vi "TransferFile.vi"(1 "Choose the Destination File Folder (Absolute Path) for AWG's files system":path, 2 "Choose the Source File (Absolute Path)":path, 4 "error in (no error)":errorcluster, 5 "ChunkSize":u32=10000000, 6 "Set File Name (with Extension)":string, 7 "VISA resource name":refnum<visa-resource-name>) -> (0 "error out":errorcluster, 3 "VISA resource name out":refnum<visa-resource-name>)   [LabVIEW 2020, in "Active Technologies AWG3000.lvlib"]
uses:
  Active Technologies AWG3000.lvlib
panel:
  # "Note: for the drive C is allowed transfer a file only to the default folder or to its subdirectories. \nNo limitation for the other drives.\nTo know the default folder, run GetDefaultDriveCFolder.vi."
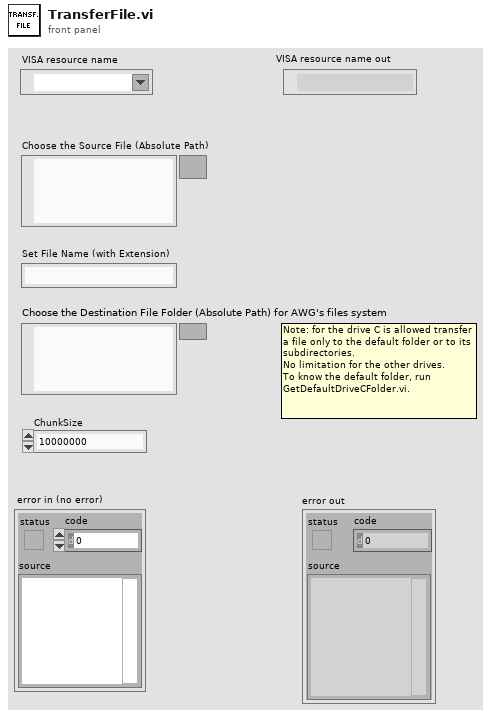
[diagram p1: front panel]
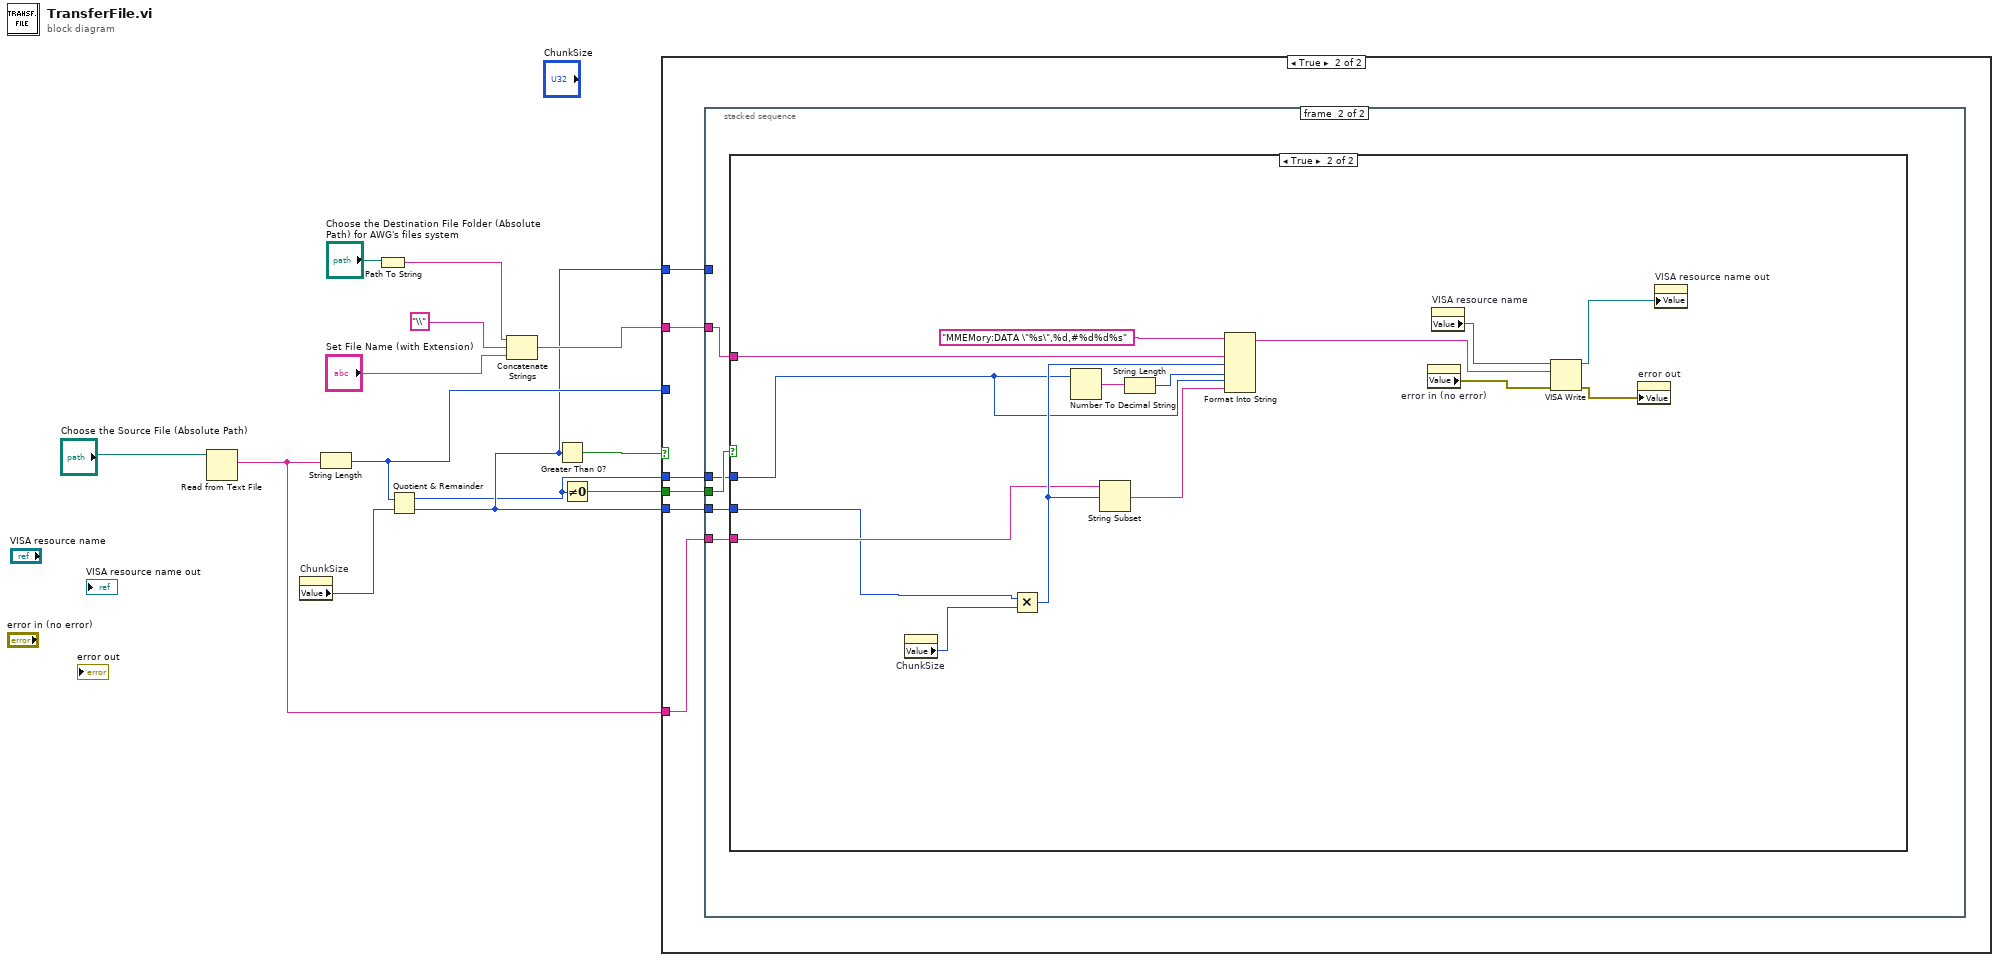
[diagram p0: block diagram]
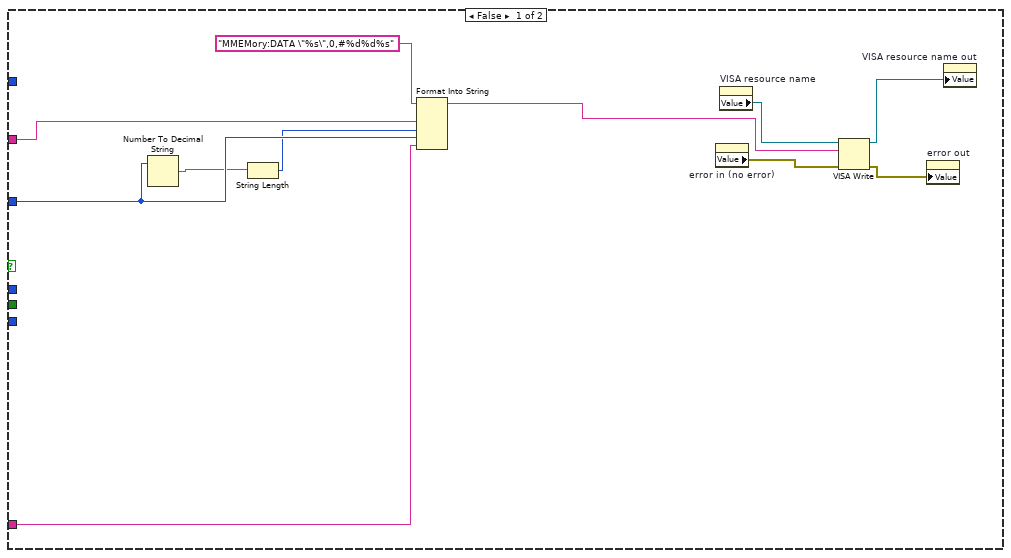
[diagram p2: hidden frame]
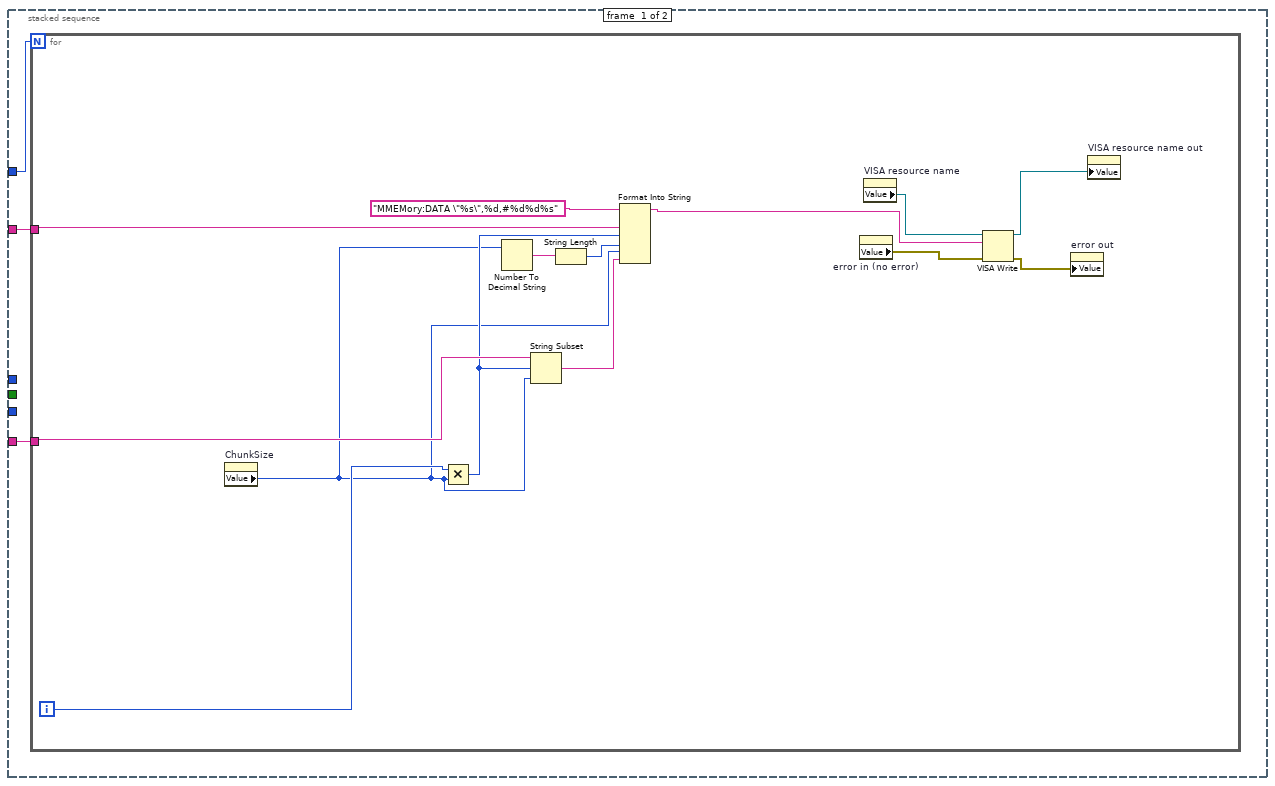
[diagram p3: hidden frame]
diagram:
  n1 = Read from Text File(file (use dialog)="Choose the Source File (Absolute Path)") -> (text=w7:string)  [unwired: 3 in, 3 out]
  n2 = property on="ChunkSize" class="DigNum (strict)"() -> ("Value"=w1:u32)  [unwired: 2 in, 2 out]
  n3 = String Length(string=w7) -> (length=w5:i32)
  n4 = Path To String(path="Choose the Destination File Folder (Absolute Path) for AWG's files system") -> (string=w12:string)
  n5 = Quotient & Remainder(x=w5, y=w1) -> (x-y*floor(x/y)=w2:u32, floor(x/y)=w3:u32)
  n6 = Concatenate Strings(w12, "\\" ("string"), "Set File Name (with Extension)") -> (w8:string)
  n7 = Greater Than 0?(x=w3) -> (x > 0?=w6:bool)
  n8 = Not Equal To 0?(x=w2) -> (x != 0?=w4:bool)
  n9 = case shown="True" w6 {
    tunnel: w8 -> [w23 w30]
    tunnel: w7 -> [w22 w29]
    tunnel: w5 -> [w21 _]
    tunnel: w3 -> [_ w28]
    tunnel: w4 -> [_ w27]
    tunnel: w3 -> [_ w26]
    tunnel: w2 -> [_ w25]
    frame False {
      n10 = Number To Decimal String(number=w21) -> (decimal integer string=w20:string)  [unwired: 1 in]
      n11 = String Length(string=w20) -> (length=w19:i32)
      n12 = Format Into String(format string="MMEMory:DATA \"%s\",0,#%d%d%s" ("write buffer"), w23, w19, w21, w22) -> (resulting string=w14:string)  [unwired: 2 in, 1 out]
      n13 = property on="error in (no error)" class="Clust (strict)"() -> ("Value"=w17:errorcluster)  [unwired: 2 in, 2 out]
      n14 = property on="VISA resource name" class="VISAName"() -> ("Value"=w16:refnum<visa-resource-name>)  [unwired: 2 in, 2 out]
      n15 = VISA Write(VISA resource name=w16, write buffer=w14, error in (no error)=w17) -> (VISA resource name out=w15:refnum<visa-resource-name>, error out=w18:errorcluster)  [unwired: 1 out]
      n16 = property on="error out" class="Clust (strict)"("Value"=w18) -> ()  [unwired: 2 in, 2 out]
      n17 = property on="VISA resource name out" class="VISAName"("Value"=w15) -> ()  [unwired: 2 in, 2 out]
    }
    frame True {
      n18 = stacked-sequence {
        tunnel: w30 -> [w33 w48]
        tunnel: w29 -> [w32 w49]
        tunnel: w28 -> [w31 _]
        tunnel: w27 -> [_ w52]
        tunnel: w26 -> [_ w51]
        tunnel: w25 -> [_ w50]
        frame #0 {
          n19 = for {
            N: w31 -> [_]
            tunnel: w33 -> [w46]
            tunnel: w32 -> [w44]
            i -> [w43]
            n20 = property on="ChunkSize" class="DigNum (strict)"() -> ("Value"=w34:u32)  [unwired: 2 in, 2 out]
            n21 = Multiply(x=w43, y=w34) -> (x*y=w40:u32)
            n22 = Number To Decimal String(number=w34) -> (decimal integer string=w42:string)  [unwired: 1 in]
            n23 = String Subset(string=w44, offset (0)=w40, length (rest)=w34) -> (substring=w45:string)
            n24 = String Length(string=w42) -> (length=w41:i32)
            n25 = Format Into String(format string="MMEMory:DATA \"%s\",%d,#%d%d%s" ("write buffer"), w46, w40, w41, w34, w45) -> (resulting string=w35:string)  [unwired: 2 in, 1 out]
            n26 = property on="error in (no error)" class="Clust (strict)"() -> ("Value"=w38:errorcluster)  [unwired: 2 in, 2 out]
            n27 = property on="VISA resource name" class="VISAName"() -> ("Value"=w37:refnum<visa-resource-name>)  [unwired: 2 in, 2 out]
            n28 = VISA Write(VISA resource name=w37, write buffer=w35, error in (no error)=w38) -> (VISA resource name out=w36:refnum<visa-resource-name>, error out=w39:errorcluster)  [unwired: 1 out]
            n29 = property on="error out" class="Clust (strict)"("Value"=w39) -> ()  [unwired: 2 in, 2 out]
            n30 = property on="VISA resource name out" class="VISAName"("Value"=w36) -> ()  [unwired: 2 in, 2 out]
          }
        }
        frame #1 {
          n31 = case shown="True" w52 {
            tunnel: w51 -> [_ w53]
            tunnel: w50 -> [_ w57]
            tunnel: w49 -> [_ w56]
            tunnel: w48 -> [_ w55]
            frame False {
            }
            frame True {
              n32 = property on="ChunkSize" class="DigNum (strict)"() -> ("Value"=w54:u32)  [unwired: 2 in, 2 out]
              n33 = Multiply(x=w53, y=w54) -> (x*y=w63:u32)
              n34 = Number To Decimal String(number=w57) -> (decimal integer string=w65:string)  [unwired: 1 in]
              n35 = String Subset(string=w56, offset (0)=w63) -> (substring=w66:string)  [unwired: 1 in]
              n36 = String Length(string=w65) -> (length=w64:i32)
              n37 = Format Into String(format string="MMEMory:DATA \"%s\",%d,#%d%d%s" ("write buffer"), w55, w63, w64, w57, w66) -> (resulting string=w58:string)  [unwired: 2 in, 1 out]
              n38 = property on="error in (no error)" class="Clust (strict)"() -> ("Value"=w61:errorcluster)  [unwired: 2 in, 2 out]
              n39 = property on="VISA resource name" class="VISAName"() -> ("Value"=w60:refnum<visa-resource-name>)  [unwired: 2 in, 2 out]
              n40 = VISA Write(VISA resource name=w60, write buffer=w58, error in (no error)=w61) -> (VISA resource name out=w59:refnum<visa-resource-name>, error out=w62:errorcluster)  [unwired: 1 out]
              n41 = property on="error out" class="Clust (strict)"("Value"=w62) -> ()  [unwired: 2 in, 2 out]
              n42 = property on="VISA resource name out" class="VISAName"("Value"=w59) -> ()  [unwired: 2 in, 2 out]
            }
          }
        }
      }
    }
  }
